vi "TeleopwithRamps.vi"(10 "Match Info":T1={"Autonomous Elapsed Seconds"=0.0, "TeleOp Elapsed Seconds"=0.0, "Disabled Elapsed Seconds"=0.0, "Visited Autonomous"=FALSE, "Visited TeleOp"=FALSE, "Visited Disabled"=FALSE, "Autonomous Settings"={"Autonomous Style"=enum."Independent", "VI Refnum"=refnum}}, 11 "Call Context":T2) -> ()   [LabVIEW 2017]
doc: "This VI is called for each enabled TeleOp packet received from the DS. It is typically used to read from joysticks and other inputs and update I/O or setpoints for timed control loops. It should complete and return within 20 milliseconds or risk missing DS packets."
uses:
  <vilib>/Rock Robotics/Network Tables/NT Write Boolean Array.vi
  <vilib>/Rock Robotics/Network Tables/NT Write Numeric Array.vi
  Control 1.ctl
  <vilib>/Rock Robotics/WPI/DriverStation/WPI_DriverStationMatch Info.ctl
  <vilib>/Rock Robotics/WPI/DriverStation/WPI_DriverStationDerivedRobotMode.ctl
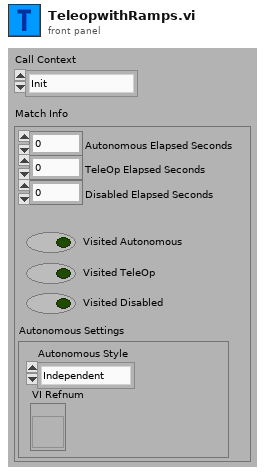
[diagram p1: front panel]
types:
  T1 = typedef "WPI_DriverStationMatch Info.ctl" = cluster{"Autonomous Elapsed Seconds":dbl, "TeleOp Elapsed Seconds":dbl, "Disabled Elapsed Seconds":dbl, "Visited Autonomous":bool, "Visited TeleOp":bool, "Visited Disabled":bool, "Autonomous Settings":cluster{"Autonomous Style":enum16{"Iterative", "Independent"}, "VI Refnum":refnum<vi>}}
  T2 = typedef "WPI_DriverStationDerivedRobotMode.ctl" = enum16{"Init", "Execute", "Stop"}
  T3 = typedef "Control 1.ctl" = enum16{"folded", "expanded"}
  T4 = typedef "WPI_JoystickDevRef.ctl" = cluster{"Device":T5}
  T5 = typedef "WPI_JoystickDeviceEnum.ctl" = enum16{"USB 0", "USB 1", "USB 2", "USB 3", "USB 4", "USB 5"}
  T6 = typedef "Command Status Info.ctl" = cluster{"Name":string, "Status":T7, "notifier out":T8}
  T7 = typedef "Completion Status.ctl" = enum16{"Successful", "Aborted", "Incomplete"}
  T8 = typedef "Completion Notifier.ctl" = refnum<notifier>
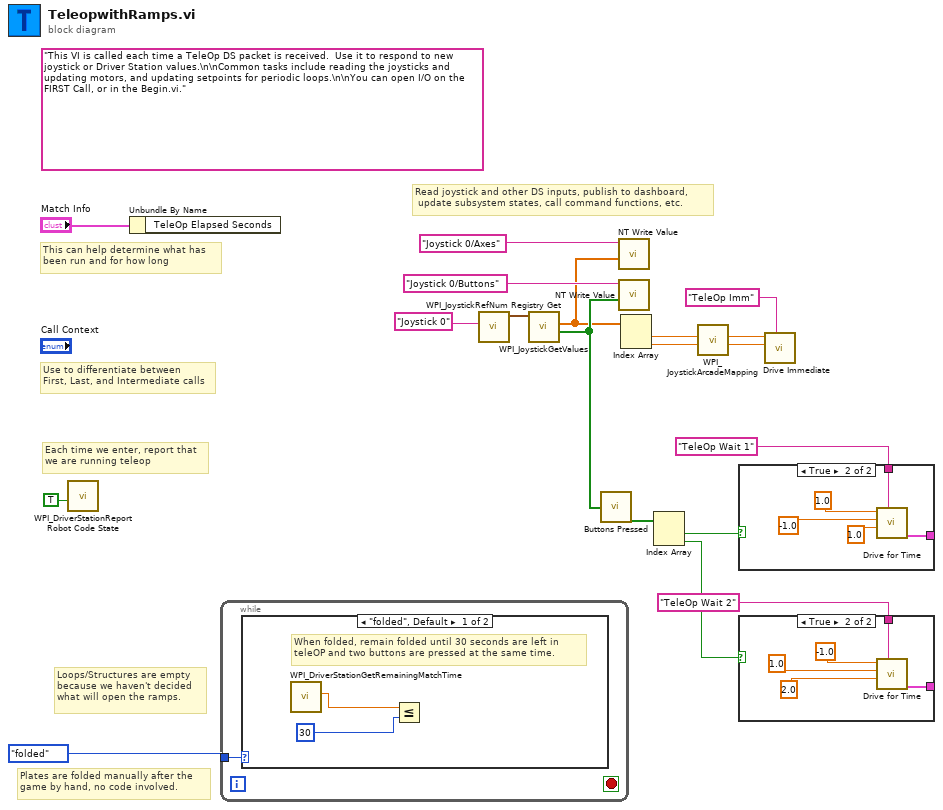
[diagram p0: block diagram]
diagram:
  (unwired) "This VI is called each time a TeleOp DS packet is received.  Use it to respond to new joystick or Driver Station values.\n\nCommon tasks include reading the joysticks and updating motors, and updating setpoints for periodic loops.\n\nYou can open I/O on the FIRST Call, or in the Begin.vi."
  # "Loops/Structures are empty\nbecause we haven't decided\nwhat will open the ramps."
  # "Plates are folded manually after the \ngame by hand, no code involved."
  # "Read joystick and other DS inputs, publish to dashboard,\n update subsystem states, call command functions, etc."
  # "Each time we enter, report that\nwe are running teleop"
  # "Use to differentiate between\nFirst, Last, and Intermediate calls"
  # "This can help determine what has\nbeen run and for how long"
  n1 = call <vilib>:"WPI_DriverStationReport Robot Code State.vi"("TeleOp"=TRUE ("Autonomous")) -> ()  [unwired: 10 in, 1 out]
  n2 = Unbundle By Name("Match Info") -> ()  [unwired: 1 out]
  n3 = while {
    tunnel: Control_1."folded" -> [w20]
    stop <- _ stop-if-true
    n4 = case shown="\"folded\", Default" w20 {
      frame "folded", Default {
        # "When folded, remain folded until 30 seconds are left in \nteleOP and two buttons are pressed at the same time."
        n5 = call <vilib>:"WPI_DriverStationGetRemainingMatchTime.vi"() -> ("Match Time(s)"=w22:sgl)  [unwired: 10 in, 1 out]
        n6 = Less Or Equal?(x=w22, y=30) -> ()  [unwired: 1 out]
      }
      frame "expanded" {
        # "If expanded, remain expanded."
      }
    }
  }
  n7 = call <vilib>:"WPI_JoystickRefNum Registry Get.vi"("refnum name"="Joystick 0") -> ("JoystickDevRef"=w16:T4)  [unwired: 1 in, 9 out]
  n8 = call <vilib>:"WPI_JoystickGetValues.vi"("JoystickDevRef"=w16) -> ("Buttons"=w4:bool[], "Axes"=w3:dbl[])  [unwired: 6 in, 3 out]
  n9 = call "Buttons Pressed.vi"("Button Values"=w4) -> ("Button Presses"=w12:bool[])
  n10 = call-poly <vilib>:"NT Write Value.vi"("Numeric Array"=w3, "Name"="Joystick 0/Axes") -> ()  [unwired: 9 in, 1 out]
  n11 = call-poly <vilib>:"NT Write Value.vi"("Boolean Array"=w4, "Name"="Joystick 0/Buttons") -> ()  [unwired: 9 in, 1 out]
  n12 = Index Array(array=w3) -> (element #1=w7:dbl, element #2=w6:dbl)  [unwired: 2 in]
  n13 = Index Array(array=w12) -> (element #1=w11:bool, element #2=w10:bool)  [unwired: 2 in]
  n14 = call <vilib>:"WPI_JoystickArcadeMapping.vi"("Y axis value"=w6, "X axis value"=w7) -> ("Right Motor Value"=w8:dbl, "Left Motor Value"=w9:dbl)  [unwired: 8 in]
  n15 = case shown="True" w11 {
    tunnel: [_ w26] -> _
    tunnel: "TeleOp Wait 1" ("Description") -> [_ w25]
    frame False {
    }
    frame True {
      n16 = call "Drive for Time.vi"("Description"=w25, "Seconds"=1.0, "Right Speed"=-1.0, "Left Speed"=1.0) -> ("Command Info Out"=w26:T6)  [unwired: 6 in, 1 out]
    }
  }
  n17 = case shown="True" w10 {
    tunnel: [_ w30] -> _
    tunnel: "TeleOp Wait 2" ("Description") -> [_ w29]
    frame False {
    }
    frame True {
      n18 = call "Drive for Time.vi"("Description"=w29, "Seconds"=2.0, "Right Speed"=1.0, "Left Speed"=-1.0) -> ("Command Info Out"=w30:T6)  [unwired: 6 in, 1 out]
    }
  }
  n19 = call "Drive Immediate.vi"("Description"="TeleOp Imm", "Right Setpoint"=w8, "Left Setpoint"=w9) -> ()  [unwired: 8 in, 1 out]
